vi "Read Single Point.vi"(8 "error in (no error)":errorcluster, 11 "PXI 4070 in":refnum<class "PXI 4070.lvclass">) -> (0 "error out":errorcluster, 2 "Measurement":dbl, 3 "PXI 4070 out":refnum<class "PXI 4070.lvclass">)   [LabVIEW 2016, in "PXI 4070.lvclass"]
uses:
  PXI 4070.lvclass
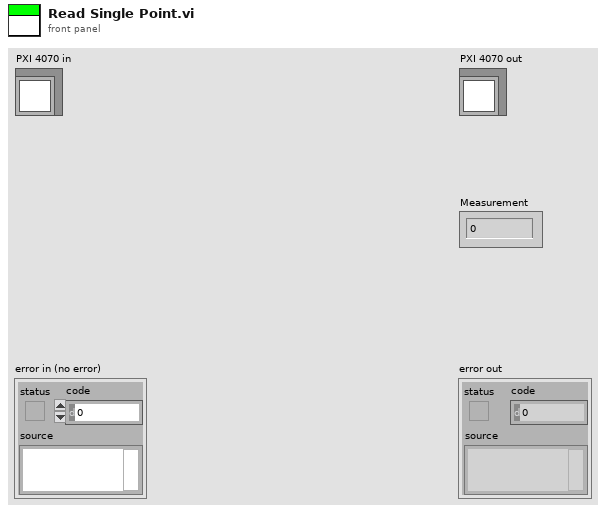
[diagram p1: front panel]
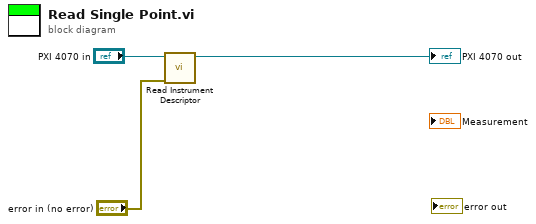
[diagram p0: block diagram]
diagram:
  n1 = call "Read Instrument Descriptor.vi"("error in (no error)"="error in (no error)", "PXI 4070 in"="PXI 4070 in") -> ("PXI 4070 out"=→"PXI 4070 out":refnum<class "PXI 4070.lvclass">)  [unwired: 7 in, 2 out]
